vi "Control Monitor.vi"(9 "Trigger Signal":bool, 10 "LED Array":dbl[](array[numeric]), 11 "Actuation Array":bool[](array[boolean])) -> ()   [LabVIEW 2024]
doc: "Dialog for selecting user specified settings."
panel:
  out "BBFuel":bool
  out "BBLOX":bool
  out "LED 16":bool
  out "LED 15":bool
  out "LED 14":bool
  out "LED 13":bool
  out "LED 12":bool
  out "LED 11":bool
  out "LED 10":bool
  out "LED 9":bool
  out "LED 8":bool
  out "LED 7":bool
  out "LED 6":bool
  out "LED 5":bool
  out "LED 4":bool
  out "LED 3":bool
  out "LED 2":bool
  out "LED 1":bool
  out "Switch 16":bool
  out "Switch 15":bool
  out "Switch 14":bool
  out "Switch 13":bool
  out "Switch 12":bool
  out "Switch 11":bool
  out "Switch 10":bool
  out "Switch 9":bool
  out "Switch 8":bool
  out "Switch 5":bool
  out "Switch 4":bool
  out "Switch 3":bool
  out "Switch 2":bool
  out "Switch 1":bool
  # "Non visible portion of dialog (needed for connector pane)."
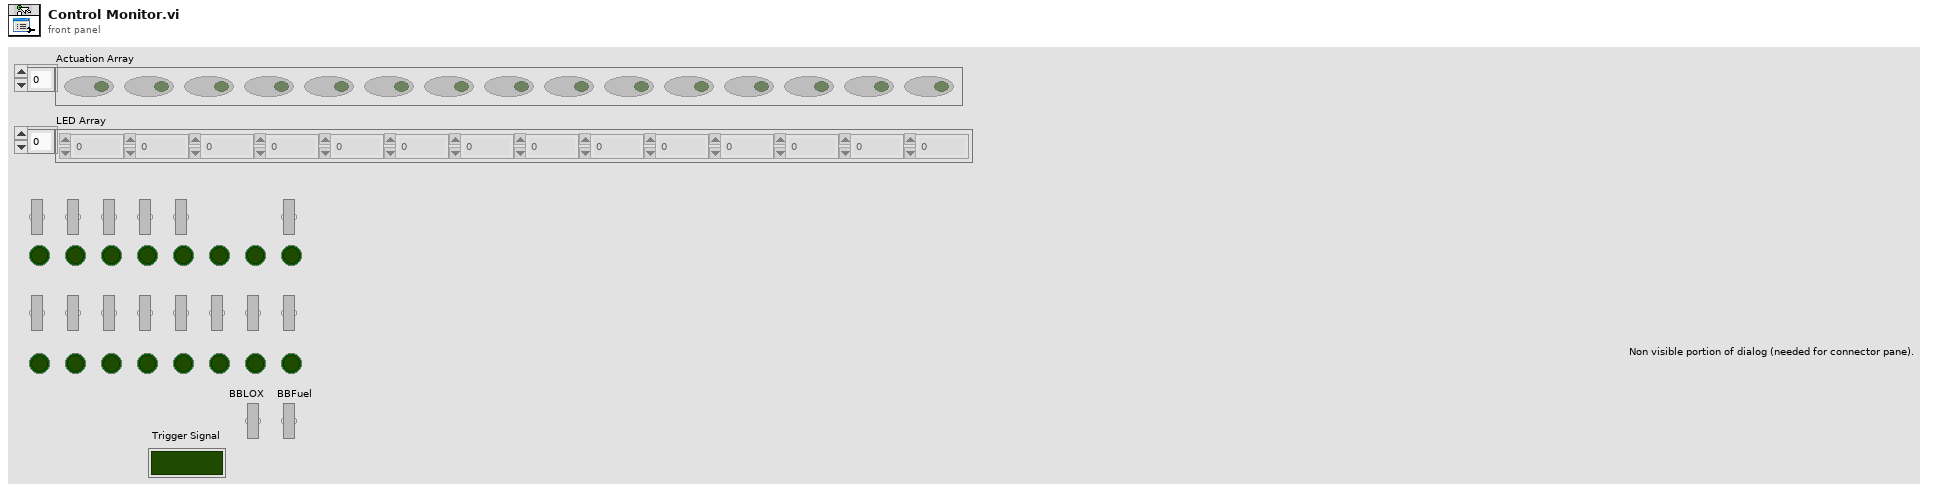
[diagram p1: front panel]
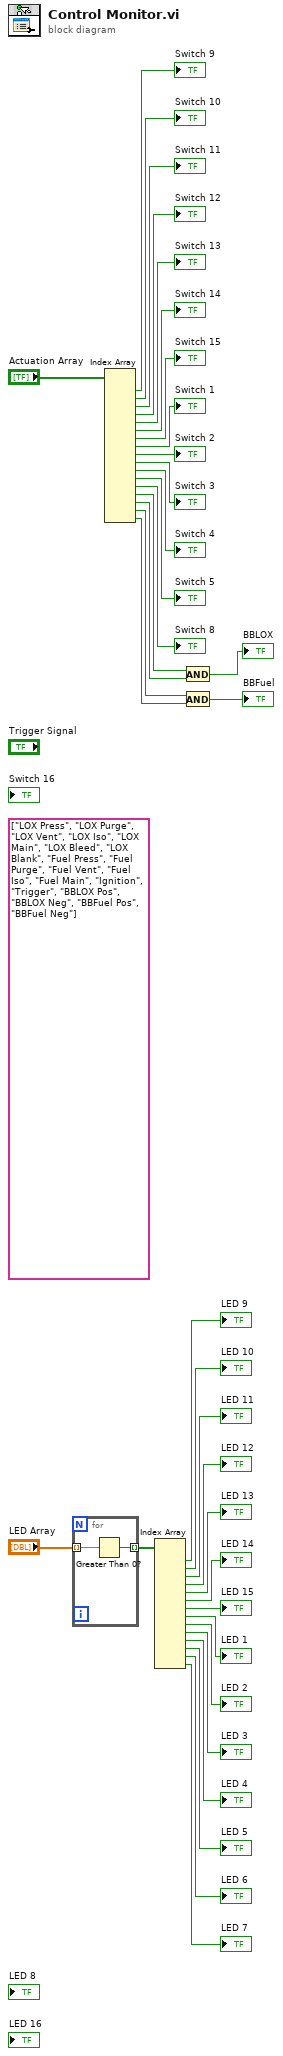
[diagram p0: block diagram]
diagram:
  (unwired) string[] ["LOX Press", "LOX Purge", "LOX Vent", "LOX Iso", "LOX Main", "LOX Bleed", "LOX Blank", "Fuel Press", "Fuel Purge", "Fuel Vent", "Fuel Iso", "Fuel Main", "Ignition", "Trigger", "BBLOX Pos", "BBLOX Neg", "BBFuel Pos", "BBFuel Neg"]
  n1 = for {
    tunnel: [w38] -> w34 mode=indexing
    tunnel: "LED Array" -> [w37] mode=indexing
    n2 = Greater Than 0?(x=w37) -> (x > 0?=w38:bool)
  }
  n3 = Index Array(array="Actuation Array") -> (element #1=→"Switch 9":bool, element #2=→"Switch 10":bool, element #3=→"Switch 11":bool, element #4=→"Switch 12":bool, element #5=→"Switch 13":bool, element #6=→"Switch 14":bool, element #7=→"Switch 15":bool, element #8=→"Switch 1":bool, element #9=→"Switch 2":bool, element #10=→"Switch 3":bool, element #11=→"Switch 4":bool, element #12=→"Switch 5":bool, element #13=→"Switch 8":bool, element #14=w4:bool, element #15=w3:bool, element #16=w2:bool, element #17=w1:bool)  [unwired: 17 in]
  n4 = Index Array(array=w34) -> (element #1=→"LED 9":bool, element #2=→"LED 10":bool, element #3=→"LED 11":bool, element #4=→"LED 12":bool, element #5=→"LED 13":bool, element #6=→"LED 14":bool, element #7=→"LED 15":bool, element #8=→"LED 1":bool, element #9=→"LED 2":bool, element #10=→"LED 3":bool, element #11=→"LED 4":bool, element #12=→"LED 5":bool, element #13=→"LED 6":bool, element #14=→"LED 7":bool)  [unwired: 14 in]
  n5 = And(x=w4, y=w3) -> (x .and. y?=→"BBLOX":bool)
  n6 = And(x=w2, y=w1) -> (x .and. y?=→"BBFuel":bool)
